vi "_Cleanup.vi"(7 "Skip Child?":bool, 8 "error in (no error)":errorcluster, 11 "Joystick in":refnum<class "Joystick.lvclass">) -> (0 "error out":errorcluster)   [LabVIEW 2020, in "Joystick.lvlib" / "Joystick.lvclass"]
uses:
  Joystick.lvclass
  Joystick.lvclass/Joystick.ctl
  <vilib>/Utility/inputDevices.llb/closeJoystick.vi
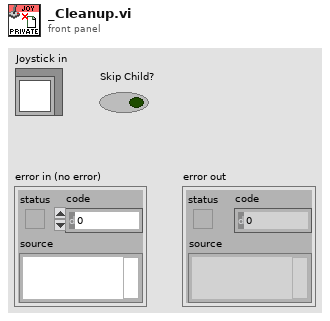
[diagram p1: front panel]
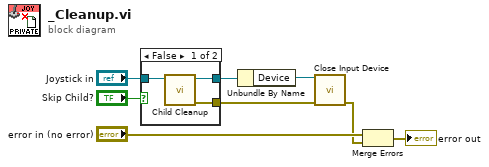
[diagram p0: block diagram]
diagram:
  n1 = case shown="False" "Skip Child?" {
    tunnel: "Joystick in" -> [w11 w12]
    tunnel: [w10 w12] -> w6
    tunnel: [w9 _] -> w4
    frame False {
      n2 = call-dynamic "Child Cleanup.vi"("Joystick in"=w11) -> ("error out"=w9:errorcluster, "Joystick out"=w10:refnum<class "Joystick.lvclass">)  [unwired: 9 in]
    }
    frame True {
    }
  }
  n3 = Unbundle By Name(w6) -> ("Device"=w5:refnum<k1>)
  n4 = call-poly <vilib>:"Close Input Device.vi"("error in (no error)"=w4, "device ID"=w5) -> ("error out"=w2:errorcluster)  [unwired: 8 in]
  n5 = Merge Errors("error in (no error)", w2) -> (→"error out":errorcluster)
